vi "MouseclickAdjustView.vi"(10 "error in (no error)":errorcluster) -> (2 "error out":errorcluster)   [LabVIEW 2014]
panel:
  out "Boolean":bool=TRUE
  in  "delay":i32=2
  in  "Y pos":i32[](array[numeric])=[497, 497, 497]
  in  "X pos":i32[](array[numeric])=[3056, 3056, 3056]
  in  "AutoItX3Lib.IAutoItX3":refnum<k7>
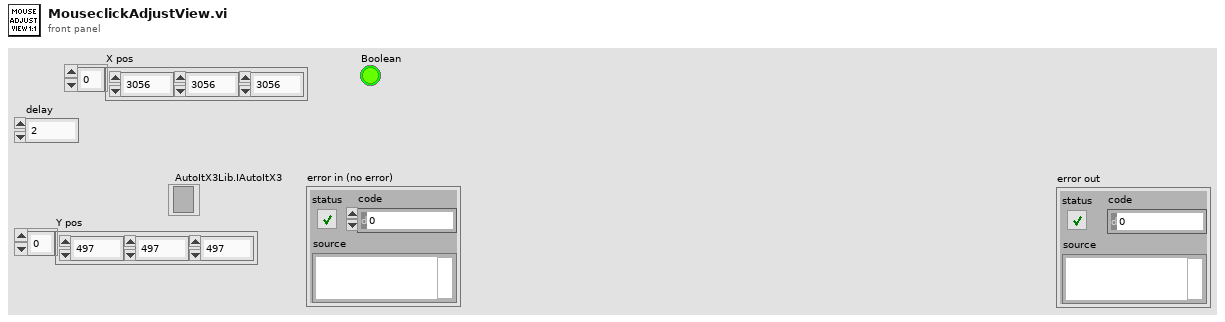
[diagram p1: front panel]
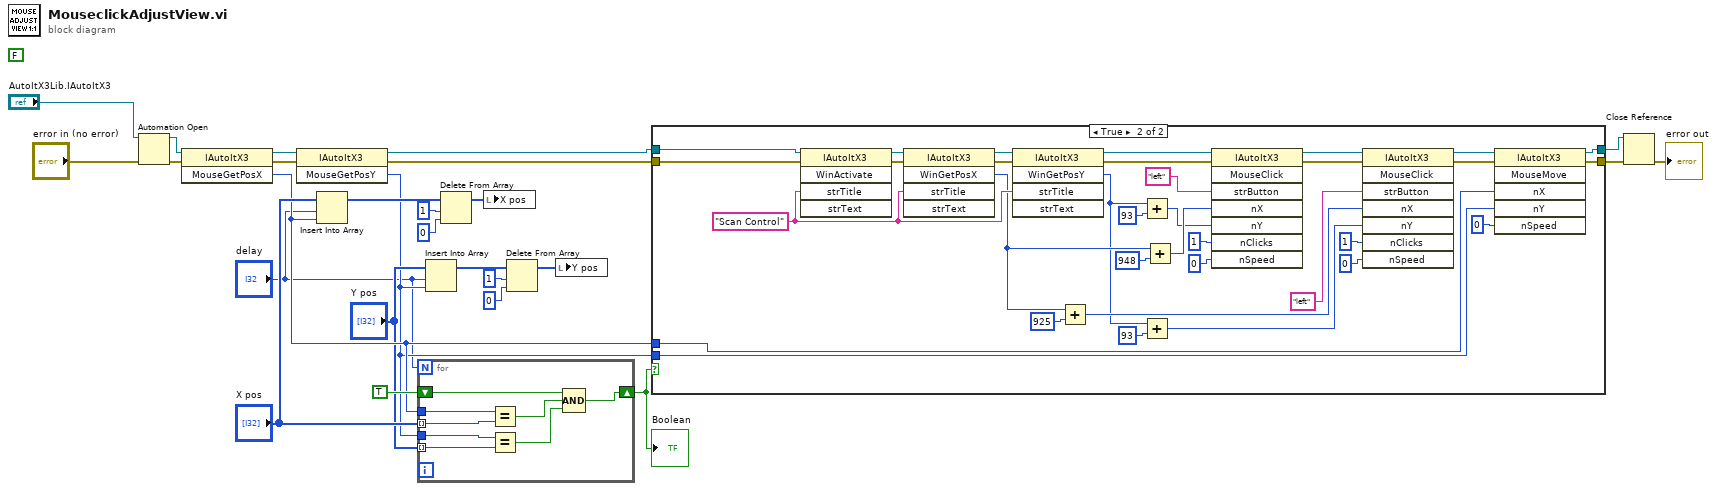
[diagram p0: block diagram]
diagram:
  (unwired) FALSE
  n1 = Automation Open(error in (no error)="error in (no error)", Automation Refnum="AutoItX3Lib.IAutoItX3") -> (Automation Refnum=w23:refnum<k7>, error out=w22:errorcluster)  [unwired: 2 in]
  n2 = invoke class="IAutoItX3" method="MouseGetPosX"(reference=w23, error in=w22) -> (reference out=w21:refnum<k7>, error out=w20:errorcluster, "MouseGetPosX"=w12:i32)  [unwired: 1 in]
  n3 = invoke class="IAutoItX3" method="MouseGetPosY"(reference=w21, error in=w20) -> (reference out=w19:refnum<k7>, error out=w18:errorcluster, "MouseGetPosY"=w2:i32)  [unwired: 1 in]
  n4 = Insert Into Array(array="X pos", index="delay", new element=w12) -> (w11:i32[])
  n5 = for {
    N: "delay" -> [_]
    tunnel: w12 -> [w34]
    tunnel: w2 -> [w33]
    shift-right: [w30] -> w14
    shift-left: TRUE -> [w29]
    tunnel: "X pos" -> [w28] mode=indexing
    tunnel: "Y pos" -> [w27] mode=indexing
    n6 = Equal?(x=w34, y=w28) -> (x = y?=w32:bool)
    n7 = Equal?(x=w33, y=w27) -> (x = y?=w31:bool)
    n8 = Compound Arithmetic op=AND(w29, w32, w31) -> (w30:bool)
  }
  "Boolean" <- w14
  n9 = Insert Into Array(array="Y pos", index="delay", new element=w2) -> (w8:i32[])
  n10 = Delete From Array(array=w11, length=1, index=0) -> (array with subset deleted=w4:i32[])  [unwired: 1 out]
  n11 = local write "X pos"(w4) -> ()
  n12 = Delete From Array(array=w8, length=1, index=0) -> (array with subset deleted=w3:i32[])  [unwired: 1 out]
  n13 = local write "Y pos"(w3) -> ()
  n14 = case shown="True" w14 {
    tunnel: w19 -> [w36 w45]
    tunnel: w18 -> [w35 w44]
    tunnel: [w36 w42] -> w17
    tunnel: [w35 w41] -> w16
    tunnel: w12 -> [_ w39]
    tunnel: w2 -> [_ w38]
    frame False {
    }
    frame True {
      w66 = "Scan Control" ("strTitle")
      n15 = invoke class="IAutoItX3" method="WinActivate"(reference=w45, error in=w44, "strTitle"=w66) -> (reference out=w70:refnum<k7>, error out=w69:errorcluster)  [unwired: 2 in, 3 out]
      n16 = invoke class="IAutoItX3" method="WinGetPosX"(reference=w70, error in=w69, "strTitle"=w66) -> (reference out=w68:refnum<k7>, error out=w67:errorcluster, "WinGetPosX"=w47:i32)  [unwired: 2 in, 2 out]
      n17 = invoke class="IAutoItX3" method="WinGetPosY"(reference=w68, error in=w67, "strTitle"=w66) -> (reference out=w60:refnum<k7>, error out=w59:errorcluster, "WinGetPosY"=w46:i32)  [unwired: 2 in, 2 out]
      n18 = Add(x=w47, y=925) -> (x+y=w53:i32)
      n19 = Add(x=w46, y=93) -> (x+y=w61:i32)
      n20 = Add(x=w46, y=93) -> (x+y=w52:i32)
      n21 = Add(x=w47, y=948) -> (x+y=w62:i32)
      n22 = invoke class="IAutoItX3" method="MouseClick"(reference=w60, error in=w59, "strButton"="left", "nX"=w62, "nY"=w61, "nClicks"=1, "nSpeed"=0) -> (reference out=w49:refnum<k7>, error out=w48:errorcluster)  [unwired: 1 in, 6 out]
      n23 = invoke class="IAutoItX3" method="MouseClick"(reference=w49, error in=w48, "strButton"="left", "nX"=w53, "nY"=w52, "nClicks"=1, "nSpeed"=0) -> (reference out=w43:refnum<k7>, error out=w40:errorcluster)  [unwired: 1 in, 6 out]
      n24 = invoke class="IAutoItX3" method="MouseMove"(reference=w43, error in=w40, "nX"=w39, "nY"=w38, "nSpeed"=0) -> (reference out=w42:refnum<k7>, error out=w41:errorcluster)  [unwired: 1 in, 4 out]
    }
  }
  n25 = Close Reference(reference=w17, error in (no error)=w16) -> (error out=→"error out":errorcluster)
